vi "niLvFpgaNotchCU(32-bit).vi"(0 "filter state in":T1, 1 "reset":bool, 5 "input data":i32, 7 "y(n-1) from accum":fxp<+/-,36,32>, 9 "adder in":i32, 11 "iteration":u8, 12 "in shift":i8=-1) -> (4 "filter state out":T1, 6 "state to multiply":i32, 8 "accumulator out":fxp<+/-,36,32> format="%.14g", 10 "adder out":i32, 15 "terminate":bool)   [LabVIEW 2017]
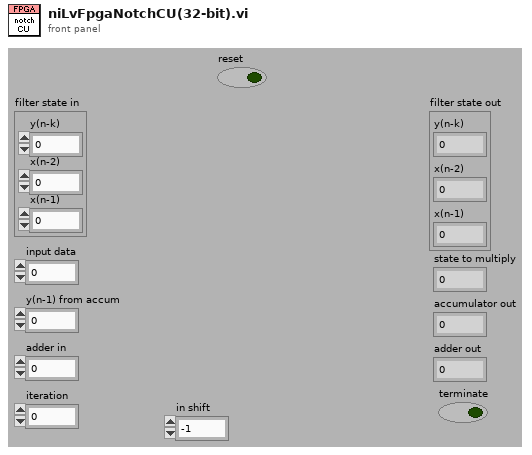
[diagram p1: front panel]
types:
  T1 = cluster{"y(n-k)":i32, "x(n-2)":i32, "x(n-1)":i32}
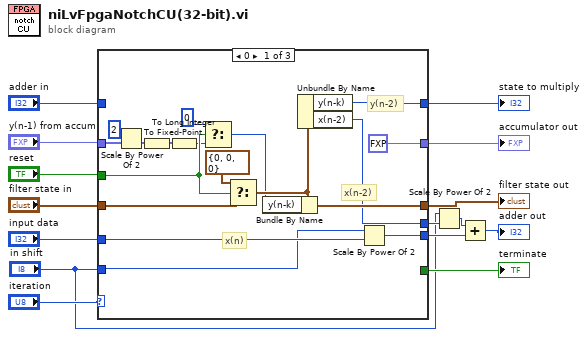
[diagram p0: block diagram]
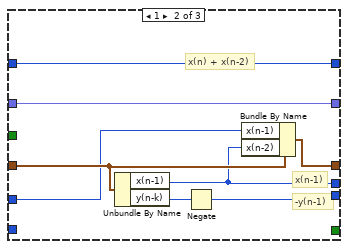
[diagram p2: hidden frame]
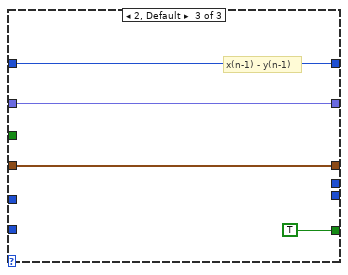
[diagram p3: hidden frame]
diagram:
  n1 = case shown="0" "iteration" {
    tunnel: [w26 w39 w45] -> w12
    tunnel: "filter state in" -> [w28 w40 w45]
    tunnel: "input data" -> [w18 w38 _]
    tunnel: [w17 w35 _] -> w6
    tunnel: "adder in" -> [_ w37 w42]
    tunnel: [w31 w37 w42] -> w11
    tunnel: "y(n-1) from accum" -> [w23 w41 w44]
    tunnel: [fxp<+/-,36,32> 0.0 ("Numeric") w41 w44] -> w8
    tunnel: [_ _ TRUE] -> w9
    tunnel: "reset" -> [w29 _ _]
    tunnel: "in shift" -> [w16 _ _]
    tunnel: [w19 w34 _] -> w3
    frame 0 {
      # "x(n)"
      # "x(n-2)"
      # "y(n-2)"
      n2 = Scale By Power Of 2(n=2, x=w23) -> (x*2^n=w22:fxp<+/-,36,32>)
      n3 = To Fixed-Point(number=w22) -> (fixed-point=w21:fxp<+/-,32,32>)  [unwired: 1 out]
      n4 = To Long Integer(number=w21) -> (32bit integer=w20:i32)
      n5 = Select(t=0, s=w29, f=w20) -> (s? t:f=w24:i32)
      n6 = Select(t=T1 {"y(n-k)"=0, "x(n-2)"=0, "x(n-1)"=0} ("filter state in"), s=w29, f=w28) -> (s? t:f=w25:T1)
      n7 = Bundle By Name(cluster=w25, "y(n-k)"=w24) -> (w26:T1)
      n8 = Unbundle By Name(w25) -> ("y(n-k)"=w31:i32, "x(n-2)"=w19:i32)
      n9 = Scale By Power Of 2(n=w16, x=w18) -> (x*2^n=w17:i32)
    }
    frame 1 {
      # "x(n) + x(n-2)"
      # "-y(n-1)"
      # "x(n-1)"
      n10 = Unbundle By Name(w40) -> ("x(n-1)"=w34:i32, "y(n-k)"=w36:i32)
      n11 = Negate(x=w36) -> (-x=w35:i32)
      n12 = Bundle By Name(cluster=w40, "x(n-1)"=w38, "x(n-2)"=w34) -> (w39:T1)
    }
    frame 2, Default {
      # "x(n-1) - y(n-1)"
    }
  }
  "filter state out" <- w12
  "state to multiply" <- w11
  "terminate" <- w9
  "accumulator out" <- w8
  n13 = Scale By Power Of 2(n="in shift", x=w3) -> (x*2^n=w1:i32)
  n14 = Add(x=w1, y=w6) -> (x+y=→"adder out":i32)
